vi "XY Graph Get Plot & Scale Strings.vi"(2 "Plot Column Header":string) -> (16 "Plot Name":string, 17 "Valid Plot Name?":bool, 18 "Scale Label":string, 19 "Valid Scale Name?":bool)   [LabVIEW 2021, in "XY Graph Add-Ons.lvlib"]
uses:
  <vilib>/Utility/error.llb/whitespace.ctl
  XY Graph/XY Graph Add-Ons.lvlib
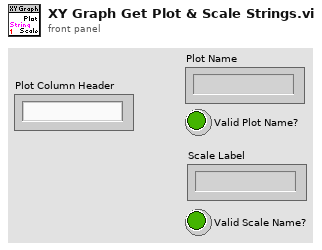
[diagram p1: front panel]
types:
  T1 = typedef "whitespace.ctl" = u16
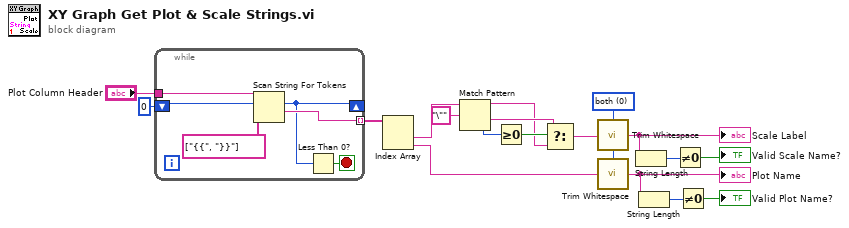
[diagram p0: block diagram]
diagram:
  w7 = T1 0 items=["both", "start of string", "end of string"] ("location (both)")
  n1 = while {
    tunnel: "Plot Column Header" -> [w23]
    shift-right: [w19] -> _
    shift-left: 0 ("offset past token") -> [w22]
    tunnel: [w20] -> w16 mode=indexing
    stop <- w21 stop-if-true
    n2 = Scan String For Tokens(6:string[] ["{{", "}}"] ("delimiters (\\s,\\t,\\r,\\n)"), 8:w22, 9:w23) -> (1:w20:string, 2:w19:i32)  [unwired: 3 in, 2 out]
    n3 = Less Than 0?(x=w19) -> (x < 0?=w21:bool)
  }
  n4 = Index Array(array=w16) -> (element #1=w15:string, element #2=w9:string)  [unwired: 2 in]
  n5 = Match Pattern(string=w15, regular expression="\"") -> (before substring=w10:string, after substring=w11:string, offset past match=w13:i32)  [unwired: 1 in, 1 out]
  n6 = Greater Or Equal To 0?(x=w13) -> (x >= 0?=w12:bool)
  n7 = Select(t=w11, s=w12, f=w10) -> (s? t:f=w8:string)
  n8 = call <vilib>:"Trim Whitespace.vi"("string"=w8, "location (both)"=w7) -> ("trimmed string"=w6:string)
  "Scale Label" <- w6
  n9 = call <vilib>:"Trim Whitespace.vi"("string"=w9, "location (both)"=w7) -> ("trimmed string"=w2:string)
  "Plot Name" <- w2
  n10 = String Length(string=w6) -> (length=w5:i32)
  n11 = String Length(string=w2) -> (length=w3:i32)
  n12 = Not Equal To 0?(x=w5) -> (x != 0?=→"Valid Scale Name?":bool)
  n13 = Not Equal To 0?(x=w3) -> (x != 0?=→"Valid Plot Name?":bool)
